vi "podGlobals_9066.vi"() -> ()   [LabVIEW 2015]
panel:
  out "Coast Time (s)":dbl
  out "Coast Timer (s)":dbl
  out "Z-Height BL (mm)":dbl
  out "Z-Height FL (mm)":dbl
  out "READY":bool
  out "Braking":bool
  out "Target Velocity (m/s)":dbl
  out "Timeout (s)":dbl
  out "Started":bool
  out "Back Brake Engaged":bool
  out "Front Brake Engaged":bool
  out "Door Open":bool
  out "Pusher Engaged":bool
  out "Z-Height BR (mm)":dbl
  out "Status":u8
  out "Progress":dbl
  out "Position (m)":dbl
  out "Velocity (m/s)":dbl
  out "Runtime (s)":dbl
  out "Battery 2 Voltage":dbl
  out "Battery 1 Voltage":dbl
  out "Acceleration (m/s^2)":dbl
  out "Battery Pressure (atm)":dbl
  out "Battery Temperature (C)":dbl
  out "Internal Pressure (atm)":dbl
  out "Internal Temperature (C)":dbl
  out "Z-Height FR (mm)":dbl
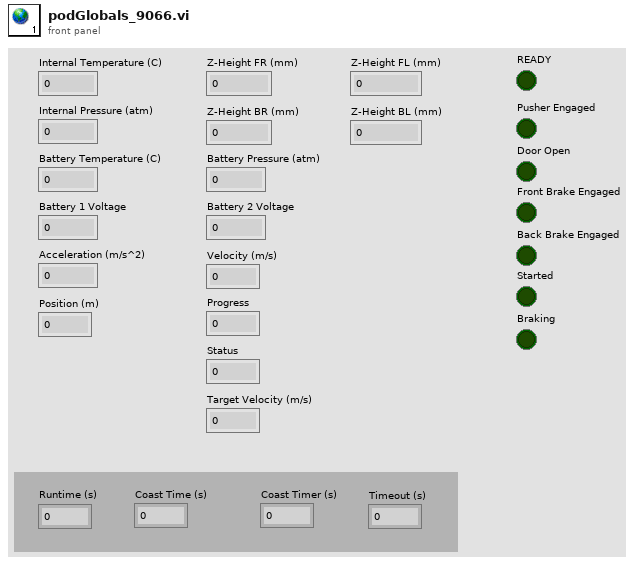
[diagram p1: front panel]
diagram:
